vi "Console_Close.vi"(8 "error in (no error)":errorcluster, 11 "Python in":T1) -> (0 "error out":errorcluster)   [LabVIEW 2022 SP3]
uses:
  PythonCtrl.ctl
  Processors.ctl
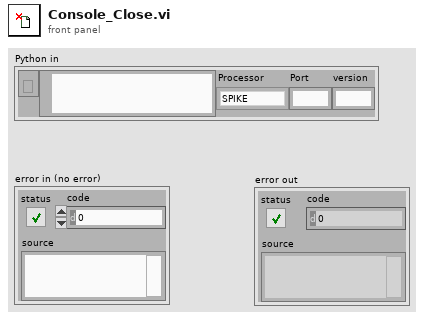
[diagram p1: front panel]
types:
  T1 = typedef "PythonCtrl.ctl" = cluster{"session":refnum<k35>, "PyPath":path, "Processor":T2, "Port":string, "version":string}
  T2 = typedef "Processors.ctl" = enum16{"SPIKE", "Pi", "Pi_ssh", "OpenMV", "Dunio"}
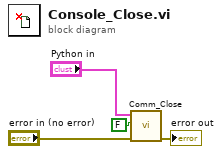
[diagram p0: block diagram]
diagram:
  n1 = call "Comm_Close.vi"("error in (no error)"="error in (no error)", "Show Err?"=FALSE, "Python in"="Python in") -> ("error out"=→"error out":errorcluster)  [unwired: 7 in, 1 out]
